vi "DSF.Shared.Configuration.Plugin.Get Transfer Group Configurations.vi"(8 "error in (no error)":errorcluster, 11 "Plugin Configuration in":refnum<class "DSF.Shared.Configuration.Plugin.lvclass">) -> (0 "error out":errorcluster, 2 "Transfer Group Configurations":refnum<class "DSF.Shared.Configuration.Transfer Group.lvclass">[](array[class]), 3 "Plugin Configuration out":refnum<class "DSF.Shared.Configuration.Plugin.lvclass">)   [LabVIEW 2016, in "DSF.Shared.lvlib" / "DSF.Shared.Configuration.Plugin.lvclass"]
uses:
  DSF.Shared.Configuration.Plugin.lvclass
  Transfer Group/DSF.Shared.Configuration.Transfer Group.lvclass
  DSF.Shared.Configuration.Plugin.lvclass/DSF.Shared.Configuration.Plugin.ctl
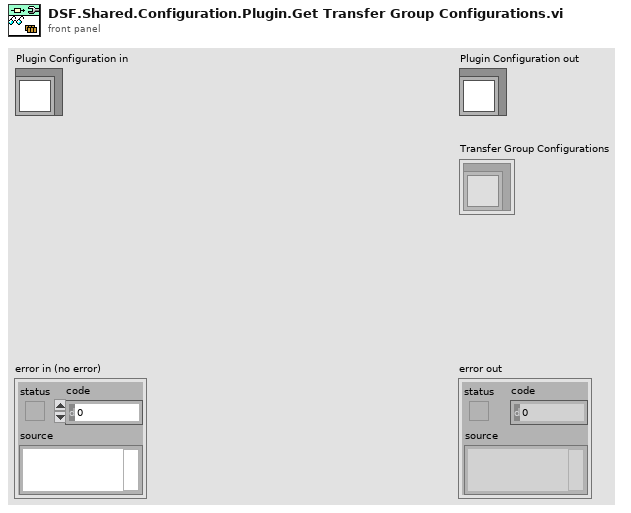
[diagram p1: front panel]
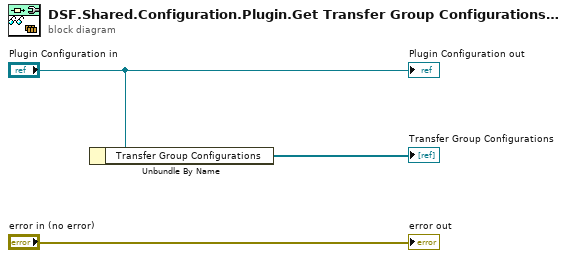
[diagram p0: block diagram]
diagram:
  n1 = Unbundle By Name("Plugin Configuration in") -> ("Transfer Group Configurations"=→"Transfer Group Configurations":refnum<class "DSF.Shared.Configuration.Transfer Group.lvclass">[])
  "error out" <- "error in (no error)"
  "Plugin Configuration out" <- "Plugin Configuration in"
